vi "Read Handle.vi"(8 "error in (no error)":errorcluster, 11 "BIO in":refnum<class "BIO.lvclass">) -> (0 "error out":errorcluster, 2 "Handle":u64, 3 "BIO out":refnum<class "BIO.lvclass">)   [LabVIEW 2013, in "OpenSSL Socket.lvlib" / "BIO.lvclass"]
uses:
  BIO.lvclass
  BIO.lvclass/BIO.ctl
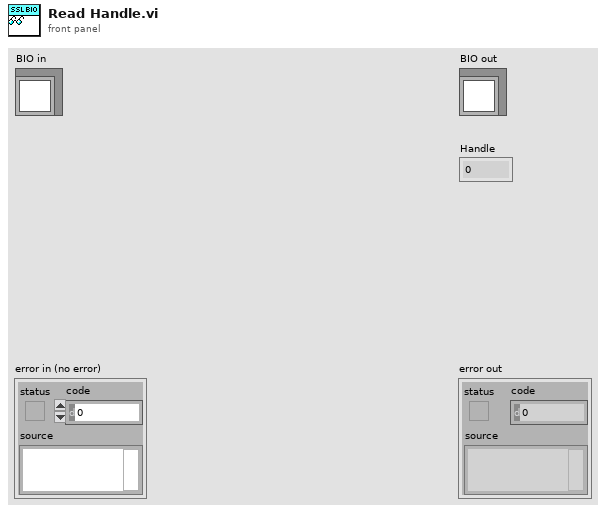
[diagram p1: front panel]
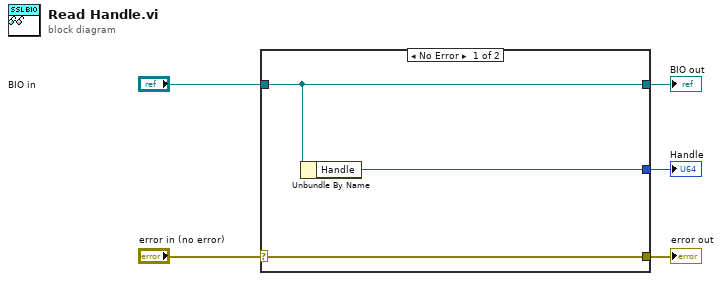
[diagram p0: block diagram]
diagram:
  n1 = case shown="No Error" "error in (no error)" {
    selector: "error in (no error)" -> [w8 w9]
    tunnel: [w8 w9] -> w4
    tunnel: [w7 w10] -> w2
    tunnel: "BIO in" -> [w7 w10]
    tunnel: [w6 _] -> w1
    frame No Error {
      n2 = Unbundle By Name(w7) -> ("Handle"=w6:u64)
    }
    frame Error {
    }
  }
  "error out" <- w4
  "BIO out" <- w2
  "Handle" <- w1
